vi "XYZ to 2D Array.vi"(7 "IntensityGraph in":refnum<vi>, 8 "2D Array Settings":T1={"x Max"=270.0, "x Min"=65.0, "x step size"=2.5, "y Max"=320.0, "y Min"=5.0, "y step size"=2.5} {"y step size" format="%#_13g"; "y Min" format="%#_13g"; "y Max" format="%#_13g"; "x step size" format="%#_13g"; "x Min" format="%#_13g"; "x Max" format="%#_13g"}, 9 "Z":dbl[](array[numeric]), 10 "Y":dbl[](array[numeric]), 11 "X":dbl[](array[numeric])) -> (1 "Y Array":dbl[](array[numeric]), 2 "X Array":dbl[](array[numeric]), 3 "2D Array out":dbl[][](array[numeric]))   [LabVIEW 2016]
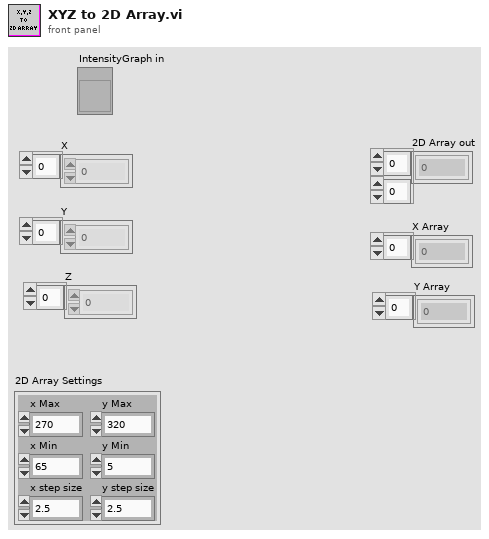
[diagram p1: front panel]
types:
  T1 = cluster{"x Max":dbl, "x Min":dbl, "x step size":dbl, "y Max":dbl, "y Min":dbl, "y step size":dbl}
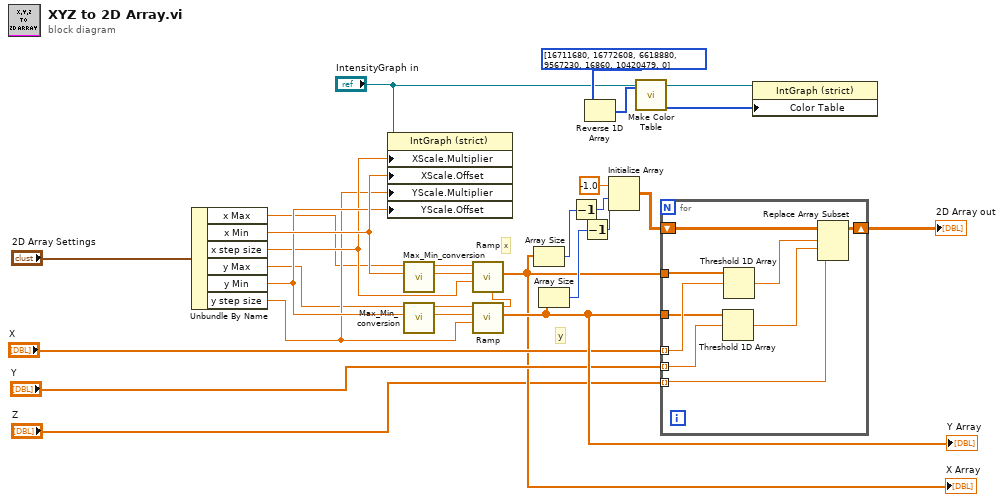
[diagram p0: block diagram]
diagram:
  # "x"
  # "y"
  n1 = Unbundle By Name("2D Array Settings") -> ("x Max"=w23:dbl, "x Min"=w28:dbl, "x step size"=w26:dbl, "y Max"=w24:dbl, "y Min"=w27:dbl, "y step size"=w25:dbl)
  n2 = property on="Property Node" class="IntGraph (strict)"(reference="IntensityGraph in", "XScale.Multiplier"=w26, "XScale.Offset"=w28, "YScale.Multiplier"=w25, "YScale.Offset"=w27) -> ()  [unwired: 1 in, 2 out]
  n3 = call <userlib>:"Max_Min_conversion.vi"("Min"=w28, "Max"=w23) -> ("offset"=w6:dbl, "Amplitude"=w5:dbl)  [unwired: 8 in]
  n4 = call <userlib>:"Max_Min_conversion.vi"("Min"=w27, "Max"=w24) -> ("offset"=w7:dbl, "Amplitude"=w8:dbl)  [unwired: 8 in]
  n5 = call <userlib>:"Ramp.vi"("step size"=w25, "offset"=w7, "amplitude"=w8) -> ("Waveform Graph"=w18:dbl[], "element"=w9:dbl)  [unwired: 6 in, 1 out]
  "Y Array" <- w18
  n6 = call <userlib>:"Ramp.vi"("i"=w9, "step size"=w26, "offset"=w6, "amplitude"=w5) -> ("Waveform Graph"=w2:dbl[])  [unwired: 5 in, 2 out]
  "X Array" <- w2
  n7 = Array Size(array=w2) -> (size(s)=w20:i32)
  n8 = Array Size(array=w18) -> (size(s)=w21:i32)
  n9 = Decrement(x=w20) -> (x-1=w16:i32)
  n10 = Decrement(x=w21) -> (x-1=w17:i32)
  n11 = Reverse 1D Array(array=u32[] [16711680, 16772608, 6618880, 9567230, 16860, 10420479, 0] ("color scale")) -> (reversed array=w11:u32[])
  n12 = Initialize Array(-1.0 ("element"), w16, w17) -> (w19:dbl[][])
  n13 = call <userlib>:"Make Color Table.vi"("Array"=w11) -> ("Color Tbl"=w12:u32[])  [unwired: 1 in, 3 out]
  n14 = for {
    tunnel: "X" -> [w36] mode=indexing
    tunnel: "Y" -> [w34] mode=indexing
    tunnel: "Z" -> [w33] mode=indexing
    tunnel: w2 -> [w37]
    tunnel: w18 -> [w35]
    shift-right: [w30] -> w15
    shift-left: w19 -> [w29]
    n15 = Threshold 1D Array(2:w34, 3:w35) -> (0:w32:dbl)  [unwired: 1 in]
    n16 = Threshold 1D Array(2:w36, 3:w37) -> (0:w31:dbl)  [unwired: 1 in]
    n17 = Replace Array Subset(array=w29, new element=w33, index (row)=w31, index (col)=w32) -> (w30:dbl[][])
  }
  "2D Array out" <- w15
  n18 = property on="Property Node" class="IntGraph (strict)"(reference="IntensityGraph in", "Color Table"=w12) -> ()  [unwired: 1 in, 2 out]
